vi "TDMS Log.vi"(8 "error in":errorcluster, 9 "Data":cluster{"Data":dbl[][]}[](array[cluster]), 10 "Channel Names":string[](array[string]), 11 "Refnum in":refnum<k34>) -> (0 "error out":errorcluster, 3 "tdms file out":refnum<k34>)   [LabVIEW 2015]
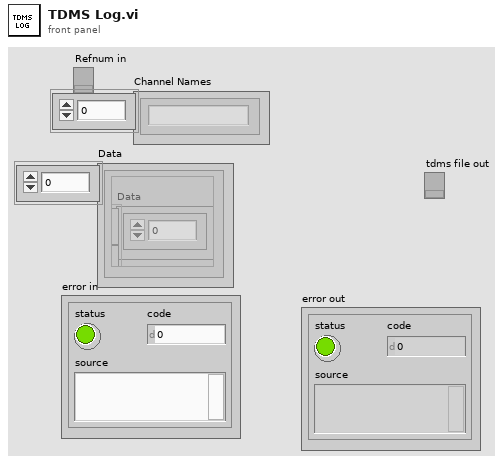
[diagram p1: front panel]
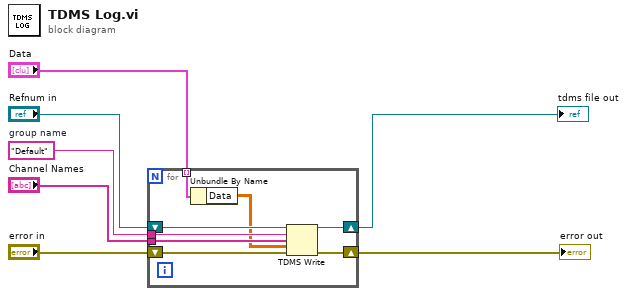
[diagram p0: block diagram]
diagram:
  w3 = "Default"  # group name
  n1 = for {
    tunnel: "Data" -> [w9] mode=indexing
    tunnel: "Channel Names" -> [w12]
    tunnel: w3 -> [w11]
    shift-right: [w10] -> w2
    shift-left: "Refnum in" -> [w15]
    shift-right: [w13] -> w5
    shift-left: "error in" -> [w14]
    n2 = Unbundle By Name(w9) -> ("Data"=w8:dbl[][])
    n3 = TDMS Write(0:w15, 5:w11, 7:w12, 9:w8, 11:w14) -> (4:w10:refnum<k34>, 15:w13:errorcluster)  [unwired: 1 in, 2 out]
  }
  "error out" <- w5
  "tdms file out" <- w2
